vi "Adapt Number Format.vi"(1 "Number In":dbl, 12 "Length":i32) -> (21 "String Out":string)   [LabVIEW 2017]
panel:
  out "error out":errorcluster
  in  "error in (no error)":errorcluster
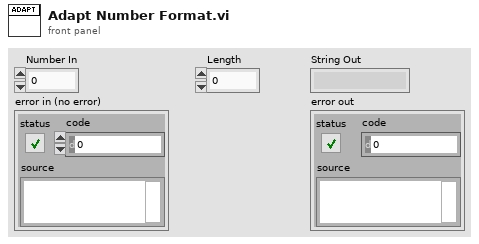
[diagram p1: front panel]
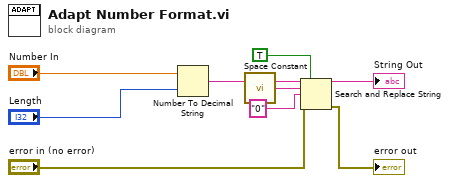
[diagram p0: block diagram]
diagram:
  n1 = Number To Decimal String(number="Number In", width (-)="Length") -> (decimal integer string=w7:string)
  n2 = call <vilib>:"Space Constant.vi"() -> ("String"=w5:string)
  n3 = Search and Replace String(replace all?=TRUE ("replace all? (F)"), input string=w7, search string=w5, replace string="0", error in="error in (no error)") -> (result string=→"String Out":string, error out=→"error out":errorcluster)  [unwired: 3 in, 2 out]
